vi "finishPrepareTriplePassPlay.vi"(8 "error in (no error)":errorcluster, 9 "Game":refnum<class "Game.lvclass">, 10 "OffensiveTeam in":refnum<class "Ally.lvclass">, 11 "PrepareTriplePassPlay in":refnum<class "PrepareTriplePassPlay.lvclass">) -> (0 "error out":errorcluster, 1 "OffensiveTeam out":refnum<class "Ally.lvclass">, 2 "finish?":bool, 3 "PrepareTriplePassPlay out":refnum<class "PrepareTriplePassPlay.lvclass">)   [LabVIEW 2021, in "PrepareTriplePassPlay.lvclass"]
uses:
  PrepareTriplePassPlay.lvclass
  Game_class/Game.lvclass
  Ally_class/Ally.lvclass
  D:/RoboIme/horie/SSL_AI/Team_class/Team.lvclass
  Referee_class/command_interpreted.ctl
  Game_class/Game.lvclass/Game.ctl
  Referee_class/Referee.lvclass/Referee.ctl
  Events_class/Events.lvclass/Events.ctl
  Team_class/Team.lvclass/Team.ctl
  Ally_class/Ally.lvclass/Ally.ctl
  Ally_class/Read PreparePassPlaysEnum.vi
  Ally_class/Write PreparePassPlaysEnum.vi
  Game_class/Read OffensiveTeam.vi
  Team_class/Read OffensivePlay Finished.vi
  Game_class/Read EventsRef.vi
  Events_class/Read ball_out.vi
  Game_class/Read Referee.vi
  Referee_class/Read command_interpreted.vi
  Referee_class/Referee.lvclass
  Events_class/Events.lvclass
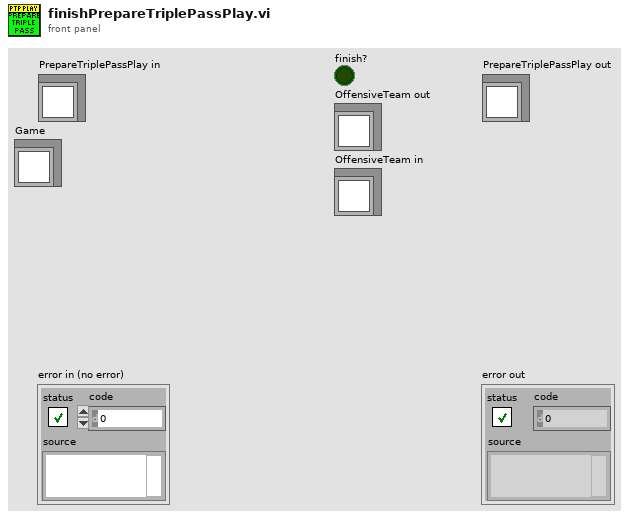
[diagram p1: front panel]
types:
  T1 = typedef "command_interpreted.ctl" = enum16{"Goal Ally", "Goal Enemy", "Ball Placement Enemy", "Ball Placement Ally", "Normal Half Time", "Extra Time  Break", "Extra Half Time", "None", "Post Game", "PKA Normal Start", "Prepare Kickoff Ally", "PKE Normal Start", "Prepare Kickoff Enemy", "Force Start", "Halt", "Timeout", "Prepare Penalty Ally", "Prepare Penalty Enemy", "PPA NormalStart", "PPE Normal Start", "Indirect Free Ally", "Direct Free Enemy", "Direct Free Ally", "Indirect Free Enemy", "Stop"}
  T2 = typedef "OffensivePlay.ctl" = enum16{"5RobotsPassGamePlay", "5PreparePassGame", "5RobotsKeeperGame", "KeeperPassToStriker", "5RobotsNormalGamePlay", "PrepareKeeperPass", "ACBPass", "ABCPass", "PrepareTriplePass", "TableWithStriker", "TableWith2ndStrikerPlay", "PrepareDoublePass", "PrepareRollToPass", "SimplePass", "PreparePass", "PassToStriker", "BallOutOfField", "PassTo2ndStriker", "StopOffensive", "Prepare Penalty Enemy", "EnemyPossessionAtEnemyField", "EnemyPossesionAtOurField", "TestPlay", "PreparePenaltyAlly", "KickPenaltyAlly", "PrepareKickoffAlly", "PrepareKickoffEnemy", "IndirectEnemy", "DirectEnemy", "PreparePassInGame1", "NormalGame", "DirectKick", "Pass", "Halt", "Timeout", "PassPlay", "PenaltyEnemy"}
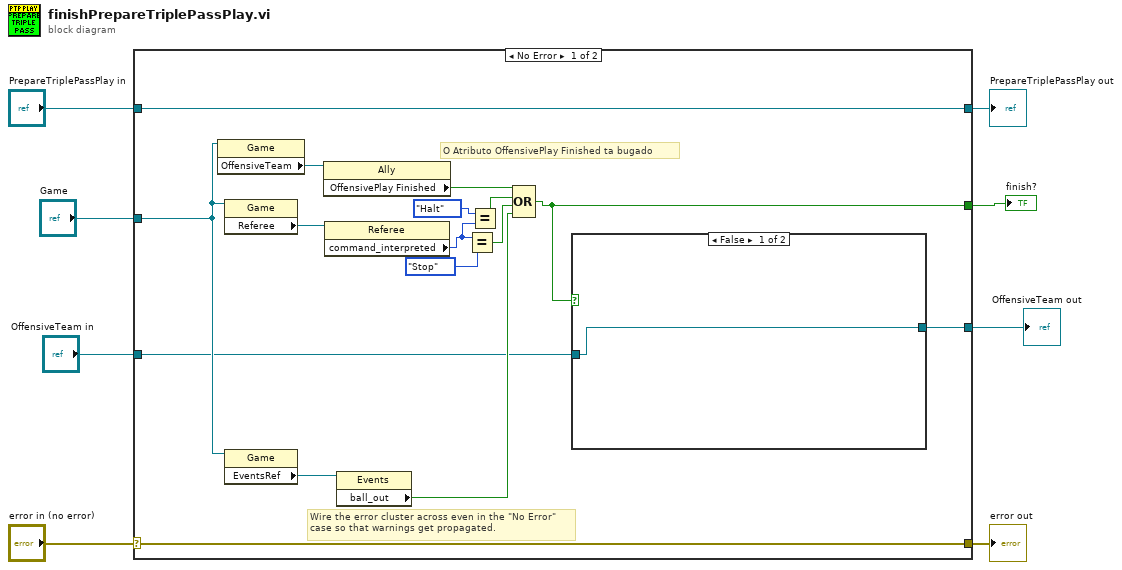
[diagram p0: block diagram]
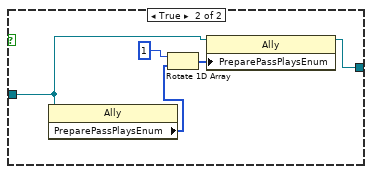
[diagram p2: hidden frame]
diagram:
  n1 = case shown="No Error" "error in (no error)" {
    selector: "error in (no error)" -> [w23 w32]
    tunnel: [w23 w32] -> w7
    tunnel: [w24 w31] -> w5
    tunnel: "PrepareTriplePassPlay in" -> [w24 w31]
    tunnel: "Game" -> [w12 _]
    tunnel: [w9 _] -> w3
    tunnel: [w11 _] -> w2
    tunnel: "OffensiveTeam in" -> [w10 _]
    frame No Error {
      # "O Atributo OffensivePlay Finished ta bugado"
      # "Wire the error cluster across even in the \"No Error\"\ncase so that warnings get propagated."
      n2 = property class="Game"(reference=w12) -> ("OffensiveTeam"=w22:refnum<class "Ally.lvclass">)  [unwired: 1 in, 2 out]
      n3 = property class="Game"(reference=w12) -> ("Referee"=w21:refnum<class "Referee.lvclass">)  [unwired: 1 in, 2 out]
      n4 = property class="Game"(reference=w12) -> ("EventsRef"=w20:refnum<class "Events.lvclass">)  [unwired: 1 in, 2 out]
      n5 = property class="Ally"(reference=w22) -> ("OffensivePlay Finished"=w13:bool)  [unwired: 1 in, 2 out]
      n6 = property class="Referee"(reference=w21) -> ("command_interpreted"=w17:T1)  [unwired: 1 in, 2 out]
      n7 = property class="Events"(reference=w20) -> ("ball_out"=w14:bool)  [unwired: 1 in, 2 out]
      n8 = Equal?(x=w17, y=command_interpreted."Stop") -> (x = y?=w19:bool)
      n9 = Equal?(x=command_interpreted."Halt" ("y"), y=w17) -> (x = y?=w15:bool)
      n10 = Compound Arithmetic op=OR(w13, w15, w19, w14) -> (w9:bool)
      n11 = case shown="False" w9 {
        tunnel: [w25 w28] -> w11
        tunnel: w10 -> [w25 w27]
        frame False {
        }
        frame True {
          n12 = property class="Ally"(reference=w27) -> ("PreparePassPlaysEnum"=w26:T2[])  [unwired: 1 in, 2 out]
          n13 = Rotate 1D Array(1:w26, 2:1 ("n")) -> (0:w29:T2[])
          n14 = property class="Ally"(reference=w27, "PreparePassPlaysEnum"=w29) -> (reference out=w28:refnum<class "Ally.lvclass">)  [unwired: 1 in, 1 out]
        }
      }
    }
    frame Error {
    }
  }
  "error out" <- w7
  "PrepareTriplePassPlay out" <- w5
  "finish?" <- w3
  "OffensiveTeam out" <- w2
